vi "Xctrl interface-Set cursors to max-min.vi"(8 "error in (no error)":errorcluster, 10 "input cluster":cluster{"X-axis max":dbl, "X-axis min":dbl}) -> (0 "error out":errorcluster)   [LabVIEW 2020]
uses:
  XGrapher.xctl
  Global variables/gl_Functional Imaging-Global variables.vi
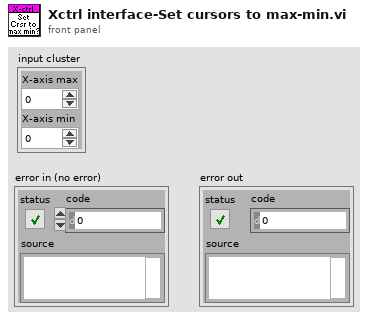
[diagram p1: front panel]
types:
  T1 = typedef "Functional Imging UI Refs.ctl" = cluster{"Menu ref":refnum<k9>, "Image control":refnum<vi>, "VI ref":refnum<vi>, "XGrapher":refnum<vi>, "Smoothing":refnum<vi>, "POI Averaging":refnum<vi>, "Normalize":refnum<vi>, "POI data points in each trial":refnum<vi>, "Channel":refnum<vi>, "Experiment data folder path":refnum<vi>, "[ROI vis]":refnum<vi>, "[Groups] visbl":T2, "Group Name":refnum<vi>, "POI index":refnum<vi>, "Trial No.":refnum<vi>, "Intensity Zoom":refnum<vi>, "Trial Cursor Enabled":refnum<vi>, "Number of Trials (ind 1)":refnum<vi>, "Number of Trials (ind 2)":refnum<vi>, "MiniScans Available":refnum<vi>, "POI Available":refnum<vi>, "Defer graph updates":refnum<vi>, "Waveform selector":refnum<vi>, "#of selected POI":refnum<vi>, "#of selected MiniScans":refnum<vi>, "#of selected groups":refnum<vi>, "Max Z-Projection":refnum<vi>, "Z-Plane Selector":refnum<vi>, "Index of miniscan point to visualise":refnum<vi>, "ROI vis. mode":refnum<vi>, "Total # of points":refnum<vi>, "Index of group clicked on":refnum<vi>, "Pane 1":refnum<vi>, "Pane 2":refnum<vi>, "Pane 3":refnum<vi>, "Pane 4":refnum<vi>, "Pane 5":refnum<vi>, "Pane 6":refnum<vi>, "Deselect all ROI":refnum<vi>, "Deselect all groups":refnum<vi>}
  T2 = typedef "Groups array referecne.ctl" = refnum<vi>
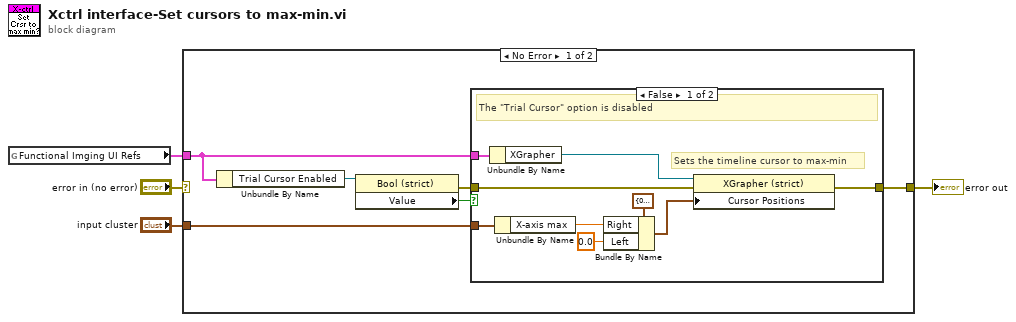
[diagram p0: block diagram]
diagram:
  n1 = global read "gl_Functional Imaging-Global variables.vi" "Functional Imging UI Refs"() -> (w1:T1)
  n2 = case shown="No Error" "error in (no error)" {
    selector: "error in (no error)" -> [_ w21]
    tunnel: [w10 w21] -> w4
    tunnel: w1 -> [w9 _]
    tunnel: "input cluster" -> [w5 _]
    frame No Error {
      n3 = Unbundle By Name(w9) -> ("Trial Cursor Enabled"=w8:refnum<vi>)
      n4 = property on="Property Node" class="Bool (strict)"(reference=w8) -> (error out=w6:errorcluster, "Value"=w7:bool)  [unwired: 1 in, 1 out]
      n5 = case shown="False" w7 {
        tunnel: [w13 w20] -> w10
        tunnel: w9 -> [w15 _]
        tunnel: w6 -> [w12 w20]
        tunnel: w5 -> [w16 _]
        frame False {
          # "Sets the timeline cursor to max-min"
          # "The \"Trial Cursor\" option is disabled"
          n6 = Unbundle By Name(w15) -> ("XGrapher"=w11:refnum<vi>)
          n7 = Unbundle By Name(w16) -> ("X-axis max"=w19:dbl)
          n8 = Bundle By Name(cluster=cluster{"Left":dbl, "Right":dbl} {"Left"=0.0, "Right"=0.0} ("Timeline Cursor Positions"), "Right"=w19, "Left"=0.0) -> (w14:cluster{"Left":dbl, "Right":dbl})
          n9 = property on="Property Node" class="XGrapher (strict)"(reference=w11, error in=w12, "Cursor Positions"=w14) -> (error out=w13:errorcluster)  [unwired: 1 out]
        }
        frame True {
          # "The \"Trial Cursor\" option is enabled"
        }
      }
    }
    frame Error {
    }
  }
  "error out" <- w4
